vi "Update Kitchen Fire and Timer.vi"(8 "error in (no error)":errorcluster, 11 "Cooker Actor in":refnum<class "Cooker Actor.lvclass">) -> (0 "error out":errorcluster, 3 "Cooker Actor out":refnum<class "Cooker Actor.lvclass">)   [LabVIEW 2024, in "Cooker Actor.lvlib" / "Cooker Actor.lvclass"]
uses:
  Cooker Actor.lvclass
  Cooker Actor.lvclass/Cooker Actor.ctl
  <vilib>/ActorFramework/Actor/Actor.lvclass
  Kitchen Actor Messages/Update Fire Msg/Update Fire Msg.lvclass
  Kitchen Actor Messages/Update Timer Msg/Update Timer Msg.lvclass
  C:/Program Files/National Instruments/LabVIEW 2024/vi.lib/ActorFramework/Actor/Actor.lvclass
  C:/Users/burakkorkmaz/Desktop/Leveling/repo/Cooker Actor/Cooker Actor/Cooker Actor.lvclass
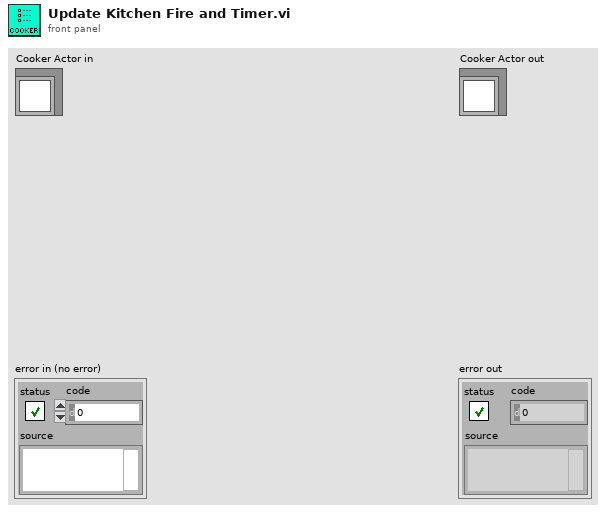
[diagram p1: front panel]
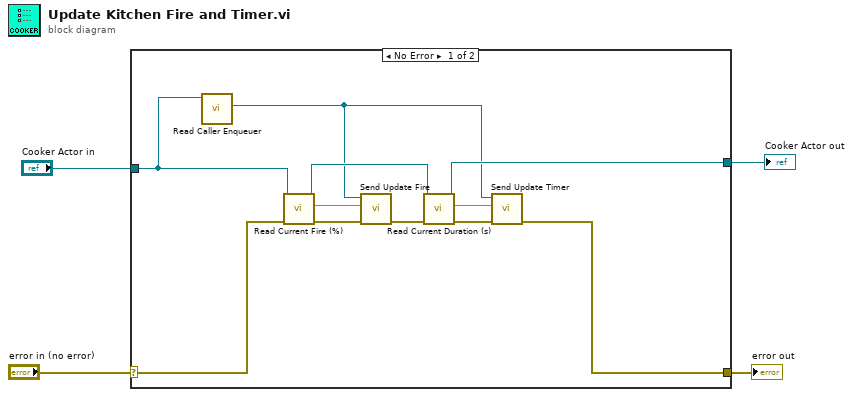
[diagram p0: block diagram]
diagram:
  n1 = case shown="No Error" "error in (no error)" {
    selector: "error in (no error)" -> [w11 w17]
    tunnel: [w15 w17] -> w3
    tunnel: [w14 w16] -> w1
    tunnel: "Cooker Actor in" -> [w13 w16]
    frame No Error {
      n2 = call <vilib>:"Read Caller Enqueuer.vi"("Actor"=w13) -> ("Caller Enqueuer"=w6:refnum<class "Message Enqueuer.lvclass">)  [unwired: 10 in]
      n3 = call-dynamic "Read Current Fire (%).vi"("error in (no error)"=w11, "Cooker Actor in"=w13) -> ("error out"=w10:errorcluster, "Current Fire (%)"=w9:dbl, "Cooker Actor out"=w12:refnum<class "Cooker Actor.lvclass">)  [unwired: 7 in]
      n4 = call "Send Update Fire.vi"("error in (no error)"=w10, "Fire (%)"=w9, "Message Enqueuer"=w6) -> ("error out"=w8:errorcluster)  [unwired: 7 in, 1 out]
      n5 = call-dynamic "Read Current Duration (s).vi"("error in (no error)"=w8, "Cooker Actor in"=w12) -> ("error out"=w7:errorcluster, "Current Duration (s)"=w5:dbl, "Cooker Actor out"=w14:refnum<class "Cooker Actor.lvclass">)  [unwired: 7 in]
      n6 = call "Send Update Timer.vi"("error in (no error)"=w7, "Timer (s)"=w5, "Message Enqueuer"=w6) -> ("error out"=w15:errorcluster)  [unwired: 7 in, 1 out]
    }
    frame Error {
    }
  }
  "error out" <- w3
  "Cooker Actor out" <- w1
